vi "MoveBaxterArms.vi"(2 "node":string, 3 "Left":T1={"e0"=0.0, "e1"=0.0, "s0"=52.0, "s1"=0.0, "w0"=0.0, "w1"=0.0, "w2"=0.0} {"w2" scale=-175.25..175.25; "w1" scale=-90.0..120.0; "w0" scale=-175.25..175.25; "e1" scale=-3.0..150.0; "e0" scale=-173.5..173.5; "s1" scale=-123.0..60.0; "s0" scale=-141.0..51.0}, 4 "Right":T1={"e0"=0.0, "e1"=0.0, "s0"=52.0, "s1"=0.0, "w0"=0.0, "w1"=0.0, "w2"=0.0} {"w2" scale=-175.25..175.25; "w1" scale=-90.0..120.0; "w0" scale=-175.25..175.25; "e1" scale=-3.0..150.0; "e0" scale=-173.5..173.5; "s1" scale=-123.0..60.0; "s0" scale=-141.0..51.0}, 6 "error in":errorcluster) -> (5 "error out":errorcluster)   [LabVIEW 2013]
doc: "This VI moves both the Baxter arms to a given position."
uses:
  ROS/Code/JointPositions.ctl
  ROS/Code/SubVIs/BaxterSide.ctl
  Command_Joint_Angles_cluster.vi
panel:
  # "If Stop Cont is set to true, the server will\nstop continuously writing"
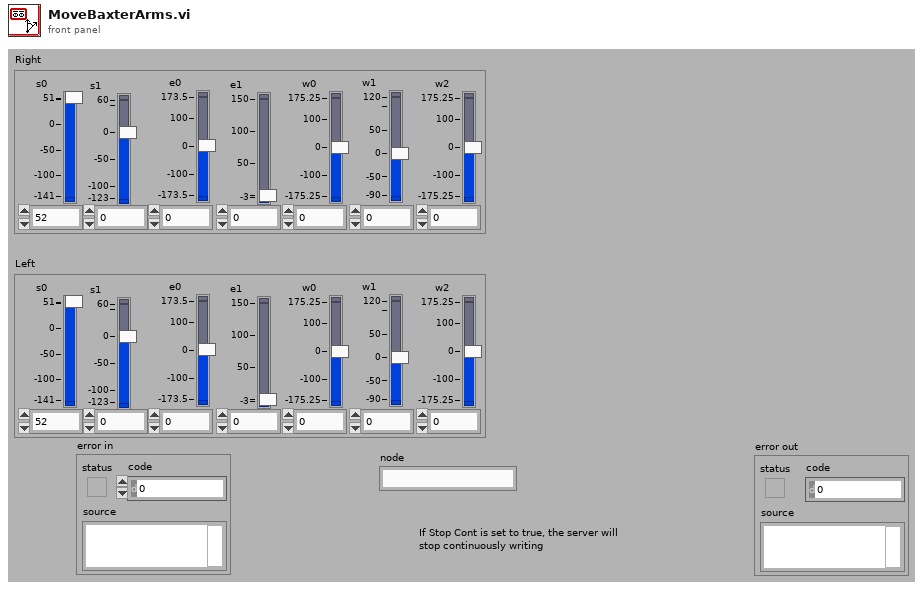
[diagram p1: front panel]
types:
  T1 = typedef "JointPositions.ctl" = cluster{"e0":dbl, "e1":dbl, "s0":dbl, "s1":dbl, "w0":dbl, "w1":dbl, "w2":dbl}
  T2 = typedef "BaxterSide.ctl" = enum16{"left", "right"}
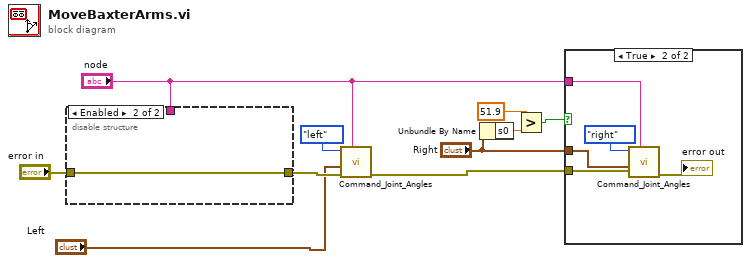
[diagram p0: block diagram]
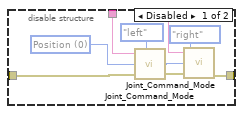
[diagram p3: hidden frame]
diagram:
  n1 = disable-structure shown="Enabled" {
    disable-tunnel: [w16 w18] -> w9
    disable-tunnel: "node" -> [w12 _]
    disable-tunnel: "error in" -> [w11 w18]
    frame Disabled {
      w15 = u8 0 items=["Position", "Velocity", "Effort"] ("Mode")
      n2 = call "Joint_Command_Mode.vi"("Side"=BaxterSide."left", "node"=w12, "Mode"=w15, "error in"=w11) -> ("error out"=w17:errorcluster)  [unwired: 2 in]
      n3 = call "Joint_Command_Mode.vi"("Side"=BaxterSide."right", "node"=w12, "Mode"=w15, "error in"=w17) -> ("error out"=w16:errorcluster)  [unwired: 2 in]
    }
    frame Enabled {
    }
  }
  n4 = call-poly "Command_Joint_Angles.vi"("node"="node", "error in"=w9, "Arm Angles (degrees)"="Left", "Side"=BaxterSide."left") -> ("error out"=w10:errorcluster)  [unwired: 5 in]
  n5 = Unbundle By Name("Right") -> ("s0"=w3:dbl)
  n6 = Greater?(x=51.9, y=w3) -> (0:w2:bool)
  n7 = case shown="True" w2 {
    tunnel: w10 -> [_ w23]
    tunnel: "node" -> [_ w21]
    tunnel: "Right" -> [_ w19]
    frame False {
    }
    frame True {
      n8 = call-poly "Command_Joint_Angles.vi"("node"=w21, "error in"=w23, "Arm Angles (degrees)"=w19, "Side"=BaxterSide."right") -> ("error out"=→"error out":errorcluster)  [unwired: 5 in]
    }
  }
